vi "Add serialNum add string header.vi"() -> ()   [LabVIEW 2021]
panel:
  out "String 2":string
  in  "String":string
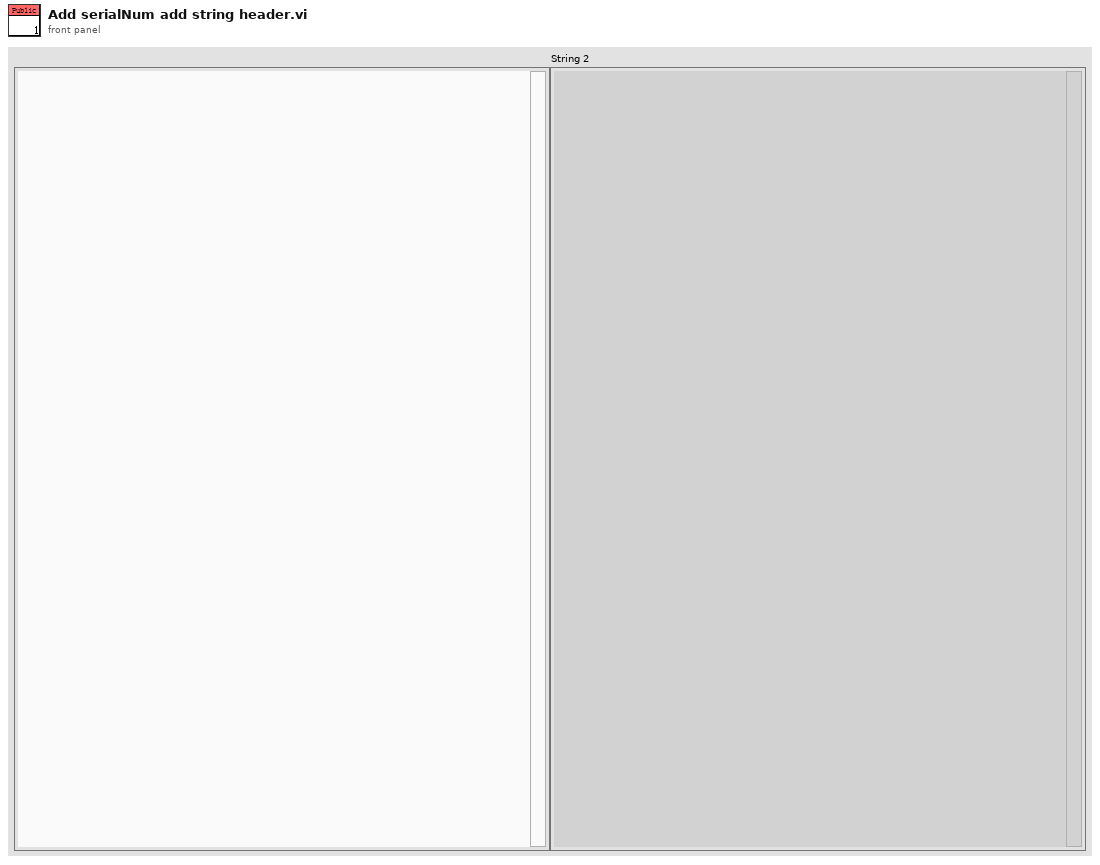
[diagram p1: front panel]
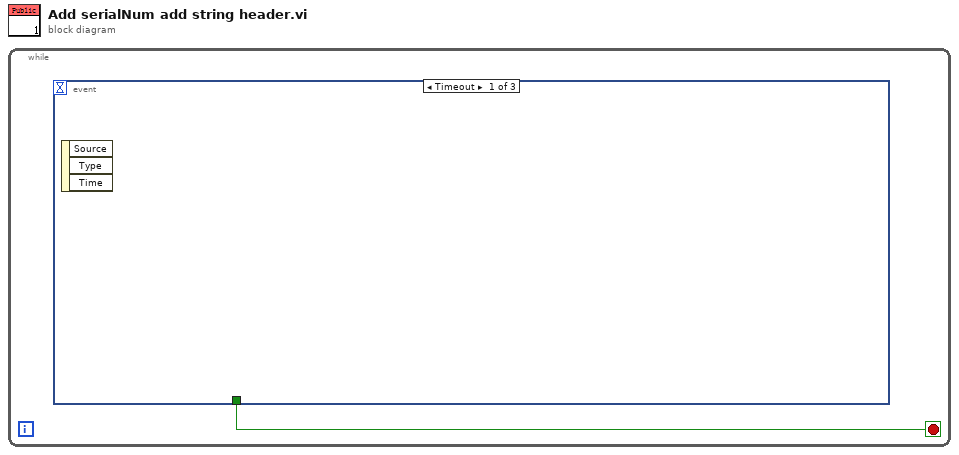
[diagram p0: block diagram]
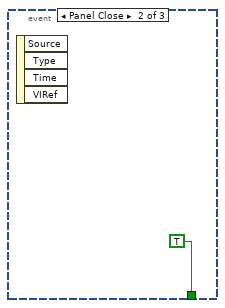
[diagram p2: hidden frame]
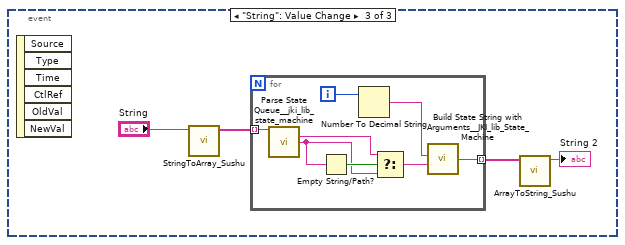
[diagram p3: hidden frame]
diagram:
  n1 = while {
    stop <- w1 stop-if-true
    n2 = event shown="[0] Timeout" {
      selector: _ -> [_ _ _]
      dyn-events: _ -> [_ _ _]
      timeout: _ -> [_ _ _]
      tunnel: [_ TRUE _] -> w1
      event Timeout {
        n3 = event-data() -> ()  [unwired: 1 in, 3 out]
      }
      event Panel Close {
        n4 = event-data() -> ()  [unwired: 1 in, 4 out]
      }
      event "String": Value Change {
        n5 = event-data() -> ()  [unwired: 1 in, 6 out]
        n6 = call <userlib>:"StringToArray_Sushu.vi"("State Queue"="String") -> ("Array"=w5:string[])  [unwired: 7 in, 3 out]
        n7 = for {
          tunnel: w5 -> [w14] mode=indexing
          tunnel: [w12] -> w4 mode=indexing
          i -> [w13]
          n8 = call <vilib>:"Parse State Queue__jki_lib_state_machine.vi"("State Queue"=w14) -> ("Current State"=w10:string, "Arguments"=w9:string)  [unwired: 11 in, 2 out]
          n9 = Empty String/Path?(string/path=w9) -> (empty?=w11:bool)
          n10 = Number To Decimal String(number=w13) -> (decimal integer string=w8:string)  [unwired: 1 in]
          n11 = Select(t=w10, s=w11, f=w9) -> (s? t:f=w7:string)
          n12 = call <vilib>:"Build State String with Arguments__JKI_lib_State_Machine.vi"("Arguments (\"\")"=w7, "State"=w8) -> ("State with Arguments"=w12:string)  [unwired: 4 in]
        }
        n13 = call <userlib>:"ArrayToString_Sushu.vi"("Array"=w4) -> ("String"=→"String 2":string)  [unwired: 10 in]
      }
    }
  }
